vi "ParseSFu.vi"(0 "data out":string) -> (5 "u1":sgl, 7 "u2":sgl)   [LabVIEW 2009]
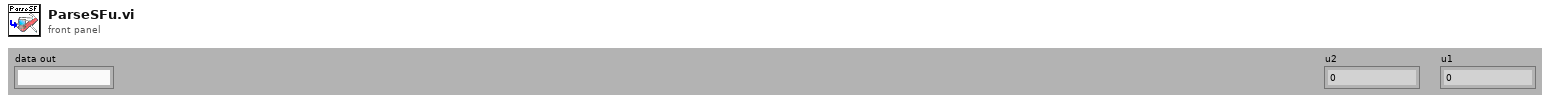
[diagram p1: front panel]
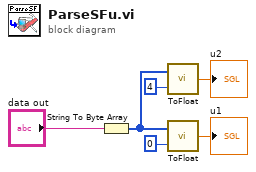
[diagram p0: block diagram]
diagram:
  n1 = String To Byte Array(string="data out") -> (unsigned byte array=w5:u8[])
  n2 = call "ToFloat.vi"("index"=4, "array"=w5) -> ("sp float"=→"u2":sgl)
  n3 = call "ToFloat.vi"("index"=0, "array"=w5) -> ("sp float"=→"u1":sgl)
